vi "AlliGator Save Local IRFs.vi"(7 "Dataset Information v1":T1, 8 "error in (no error)":errorcluster, 9 "IRF Array Time Axis":dbl[](array[numeric]), 10 "[[IRFs]]":dbl[][](array[numeric]), 11 "File Path":path) -> (0 "error out":errorcluster, 1 "Message":string)   [LabVIEW 2021, in "AlliGator IRF.lvlib"]
uses:
  AlliGator IRF.lvlib
  Files/AlliGator FLI Dataset Information v1.ctl
  <vilib>/addons/h5labview2/file/H5Fmode.ctl
  AlliGator Local IRFs HDF5 File Sections.ctl
  <vilib>/addons/h5labview2/base/lib_path.vi
  <vilib>/addons/h5labview2/base/H5Equery.vi
  <vilib>/addons/h5labview2/dataset/H5Dwrite.llb/H5Dwrite.xnode
  <vilib>/addons/h5labview2/file/H5F.lvlib
  <vilib>/addons/h5labview2/group/H5G.lvlib
  Variant/Variant.lvlib
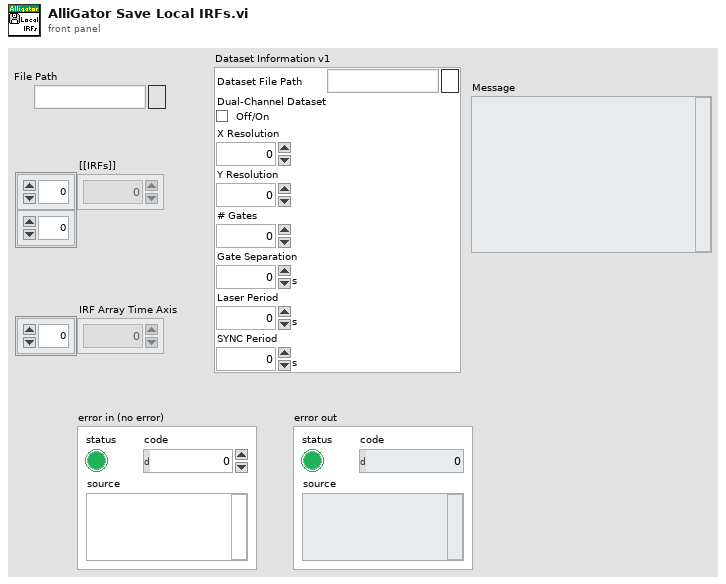
[diagram p1: front panel]
types:
  T1 = typedef "AlliGator IRF.lvlib/AlliGator FLI Dataset Information v1.ctl" = cluster{"Dataset File Path":path, "Dual-Channel Dataset":bool, "X Resolution":i32, "Y Resolution":i32, "# Gates":i32, "Gate Separation":dbl[unit], "Laser Period":dbl[unit], "SYNC Period":dbl[unit]}
  T2 = typedef "AlliGator IRF.lvlib/AlliGator Local IRFs HDF5 File Sections.ctl" = enum16{"File Information", "Dataset Information", "Local IRFs Data"}
  T3 = typedef "H5F.lvlib/H5Fmode.ctl" = enum16{"read-only", "read-write", "overwrite", "create new", "open or create"}
  T4 = typedef "hid_t.ctl" = i64
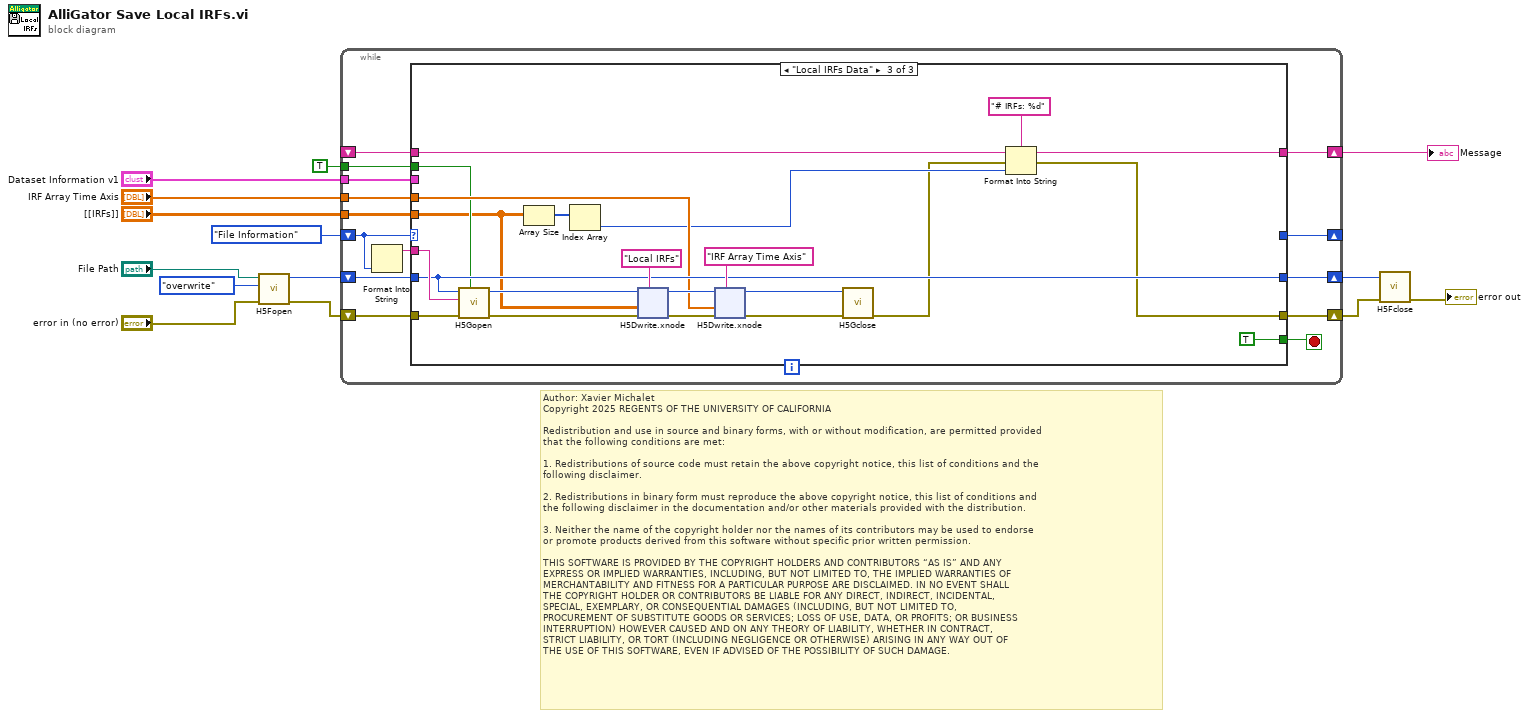
[diagram p0: block diagram]
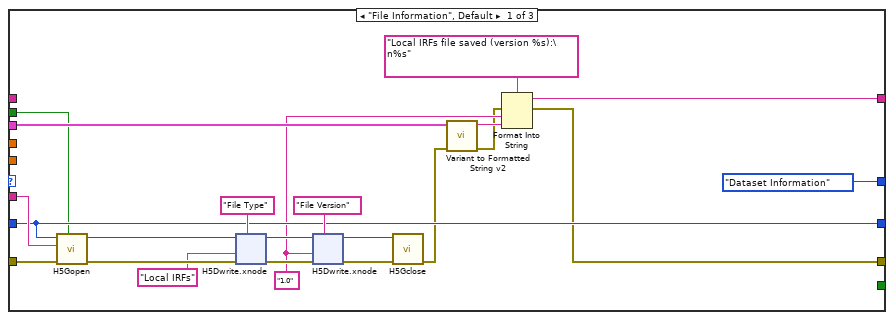
[diagram p2: hidden frame]
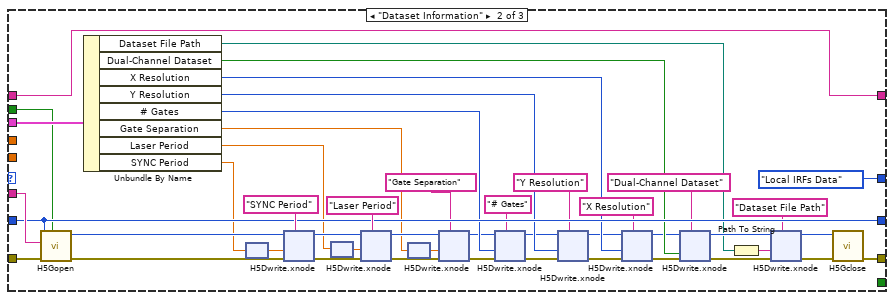
[diagram p3: hidden frame]
diagram:
  # "Author: Xavier Michalet\nCopyright 2025 REGENTS OF THE UNIVERSITY OF CALIFORNIA\n\nRedistribution and use in source and binary forms, with or without modification, are permitted provided\nthat the following conditions are met:\n\n1. Redistributions of source code must retain the above copyright notice, this list of conditions and the\nfollowing disclaimer.\n\n2. Redistributions in binary form must reproduce the above copyright notice, this list of conditions and\nthe following disclaimer in the documentation and/or other materials provided with the distribution.\n\n3. Neither the name of the copyright holder nor the names of its contributors may be used to endorse \nor promote products derived from this software without specific prior written permission.\n\nTHIS SOFTWARE IS PROVIDED BY THE COPYRIGHT HOLDERS AND CONTRIBUTORS “AS IS” AND ANY \nEXPRESS OR IMPLIED WARRANTIES, INCLUDING, BUT NOT LIMITED TO, THE IMPLIED WARRANTIES OF\nMERCHANTABILITY AND FITNESS FOR A PARTICULAR PURPOSE ARE DISCLAIMED. IN NO EVENT SHALL\nTHE COPYRIGHT HOLDER OR CONTRIBUTORS BE LIABLE FOR ANY DIRECT, INDIRECT, INCIDENTAL, \nSPECIAL, EXEMPLARY, OR CONSEQUENTIAL DAMAGES (INCLUDING, BUT NOT LIMITED TO, \nPROCUREMENT OF SUBSTITUTE GOODS OR SERVICES; LOSS OF USE, DATA, OR PROFITS; OR BUSINESS\nINTERRUPTION) HOWEVER CAUSED AND ON ANY THEORY OF LIABILITY, WHETHER IN CONTRACT, \nSTRICT LIABILITY, OR TORT (INCLUDING NEGLIGENCE OR OTHERWISE) ARISING IN ANY WAY OUT OF\nTHE USE OF THIS SOFTWARE, EVEN IF ADVISED OF THE POSSIBILITY OF SUCH DAMAGE."
  n1 = call <vilib>:"H5Fopen.vi"("error in (no error)"="error in (no error)", "mode (read-only)"=H5Fmode."overwrite", "path"="File Path") -> ("error out"=w9:errorcluster, "ref out"=w10:T4)  [unwired: 7 in]
  n2 = while {
    shift-right: [w24] -> _
    shift-left: AlliGator_Local_IRFs_HDF5_File_Sections."File Information" -> [w25]
    shift-right: [w22] -> w5
    shift-left: w10 -> [w28]
    shift-right: [w23] -> w4
    shift-left: w9 -> [w27]
    tunnel: "[[IRFs]]" -> [w20]
    tunnel: "IRF Array Time Axis" -> [w19]
    tunnel: "Dataset Information v1" -> [w18]
    shift-right: [w17] -> w2
    shift-left: _ -> [w16]
    tunnel: TRUE ("create? (F)") -> [w15]
    stop <- w21 stop-if-true
    n3 = Format Into String(w25) -> (resulting string=w26:string)  [unwired: 3 in, 1 out]
    n4 = case shown="\"Local IRFs Data\"" w25 {
      tunnel: w28 -> [w38 w124 w298]
      tunnel: w27 -> [w50 w134 w308]
      tunnel: w26 -> [w40 w127 w299]
      tunnel: [AlliGator_Local_IRFs_HDF5_File_Sections."Dataset Information" AlliGator_Local_IRFs_HDF5_File_Sections."Local IRFs Data" _] -> w24
      tunnel: [w31 w125 w287] -> w23
      tunnel: [w38 w124 w298] -> w22
      tunnel: [_ _ TRUE] -> w21
      tunnel: w20 -> [_ _ w291]
      tunnel: w19 -> [_ _ w296]
      tunnel: w18 -> [w36 w123 _]
      tunnel: [w30 w90 w293] -> w17
      tunnel: w16 -> [_ w90 w295]
      tunnel: w15 -> [w29 w89 w294]
      frame "File Information", Default {
        w35 = "1.0" ("name")
        n5 = call <vilib>:"H5Gopen.vi"("create? (F)"=w29, "error in (no error)"=w50, "name"=w40, "ref in"=w38) -> ("error out"=w48:errorcluster, "group out"=w49:T4)  [unwired: 6 in]
        n6 = xnode "H5Dwrite.xnode"("dataset name"="File Type" ("name"), "error in (no error)"=w48, "data"="Local IRFs" ("name"), "ref in"=w49) -> ("error out"=w44:errorcluster, "ref out"=w45:i64)  [unwired: 3 in, 1 out]
        n7 = xnode "H5Dwrite.xnode"("dataset name"="File Version", "error in (no error)"=w44, "data"=w35, "ref in"=w45) -> ("error out"=w42:errorcluster, "ref out"=w43:i64)  [unwired: 3 in, 1 out]
        n8 = call <vilib>:"H5Gclose.vi"("error in (no error)"=w42, "group in"=w43) -> ("error out"=w32:errorcluster)  [unwired: 9 in]
        n9 = call "Variant to Formatted String v2.vi"("error in (no error)"=w32, "Anything"=w36) -> ("error out"=w33:errorcluster, "String"=w37:string)  [unwired: 8 in]
        n10 = Format Into String(format string="Local IRFs file saved (version %s):\n%s", error in=w33, w35, w37) -> (resulting string=w30:string, error out=w31:errorcluster)  [unwired: 1 in]
      }
      frame "Dataset Information" {
        n11 = call <vilib>:"H5Gopen.vi"("create? (F)"=w89, "error in (no error)"=w134, "name"=w127, "ref in"=w124) -> ("error out"=w132:errorcluster, "group out"=w133:T4)  [unwired: 6 in]
        n12 = Unbundle By Name(w123) -> ("Dataset File Path"=w92:path, "Dual-Channel Dataset"=w103:bool, "X Resolution"=w105:i32, "Y Resolution"=w109:i32, "# Gates"=w113:i32, "Gate Separation"=w116:dbl[unit], "Laser Period"=w120:dbl[unit], "SYNC Period"=w122:dbl[unit])
        n13 = node(w122) -> (w121:dbl)
        n14 = xnode "H5Dwrite.xnode"("dataset name"="SYNC Period" ("name"), "error in (no error)"=w132, "data"=w121, "ref in"=w133) -> ("error out"=w129:errorcluster, "ref out"=w130:i64)  [unwired: 3 in, 1 out]
        n15 = node(w120) -> (w119:dbl)
        n16 = xnode "H5Dwrite.xnode"("dataset name"="Laser Period", "error in (no error)"=w129, "data"=w119, "ref in"=w130) -> ("error out"=w117:errorcluster, "ref out"=w118:i64)  [unwired: 3 in, 1 out]
        n17 = node(w116) -> (w115:dbl)
        n18 = xnode "H5Dwrite.xnode"("dataset name"="Gate Separation", "error in (no error)"=w117, "data"=w115, "ref in"=w118) -> ("error out"=w112:errorcluster, "ref out"=w99:i64)  [unwired: 3 in, 1 out]
        n19 = xnode "H5Dwrite.xnode"("dataset name"="# Gates", "error in (no error)"=w112, "data"=w113, "ref in"=w99) -> ("error out"=w110:errorcluster, "ref out"=w98:i64)  [unwired: 3 in, 1 out]
        n20 = xnode "H5Dwrite.xnode"("dataset name"="Y Resolution", "error in (no error)"=w110, "data"=w109, "ref in"=w98) -> ("error out"=w107:errorcluster, "ref out"=w97:i64)  [unwired: 3 in, 1 out]
        n21 = xnode "H5Dwrite.xnode"("dataset name"="X Resolution", "error in (no error)"=w107, "data"=w105, "ref in"=w97) -> ("error out"=w104:errorcluster, "ref out"=w96:i64)  [unwired: 3 in, 1 out]
        n22 = xnode "H5Dwrite.xnode"("dataset name"="Dual-Channel Dataset", "error in (no error)"=w104, "data"=w103, "ref in"=w96) -> ("error out"=w101:errorcluster, "ref out"=w95:i64)  [unwired: 3 in, 1 out]
        n23 = Path To String(path=w92) -> (string=w91:string)
        n24 = xnode "H5Dwrite.xnode"("dataset name"="Dataset File Path", "error in (no error)"=w101, "data"=w91, "ref in"=w95) -> ("error out"=w100:errorcluster, "ref out"=w94:i64)  [unwired: 3 in, 1 out]
        n25 = call <vilib>:"H5Gclose.vi"("error in (no error)"=w100, "group in"=w94) -> ("error out"=w125:errorcluster)  [unwired: 9 in]
      }
      frame "Local IRFs Data" {
        n26 = call <vilib>:"H5Gopen.vi"("create? (F)"=w294, "error in (no error)"=w308, "name"=w299, "ref in"=w298) -> ("error out"=w306:errorcluster, "group out"=w307:T4)  [unwired: 6 in]
        n27 = Array Size(array=w291) -> (size(s)=w290:i32[])
        n28 = Index Array(array=w290) -> (element=w289:i32)  [unwired: 1 in]
        n29 = xnode "H5Dwrite.xnode"("dataset name"="Local IRFs" ("name"), "error in (no error)"=w306, "data"=w291, "ref in"=w307) -> ("error out"=w303:errorcluster, "ref out"=w304:i64)  [unwired: 3 in, 1 out]
        n30 = xnode "H5Dwrite.xnode"("dataset name"="IRF Array Time Axis", "error in (no error)"=w303, "data"=w296, "ref in"=w304) -> ("error out"=w301:errorcluster, "ref out"=w302:i64)  [unwired: 3 in, 1 out]
        n31 = call <vilib>:"H5Gclose.vi"("error in (no error)"=w301, "group in"=w302) -> ("error out"=w288:errorcluster)  [unwired: 9 in]
        n32 = Format Into String(format string="# IRFs: %d", initial string=w295, error in=w288, w289) -> (resulting string=w293:string, error out=w287:errorcluster)
      }
    }
  }
  "Message" <- w2
  n33 = call <vilib>:"H5Fclose.vi"("error in (no error)"=w4, "ref"=w5) -> ("error out"=→"error out":errorcluster)  [unwired: 9 in]
